vi "Transmitter_Monokrom_Mei - Copy.vi"() -> ()   [LabVIEW 2018]
uses:
  <vilib>/picture/picture.llb/imagedata.ctl
  <instrlib>/niUSRP/niUSRP Write Tx Data (CDB Cluster).vi
panel:
  out "size(s) 6":i32[](array[numeric])
  out "size(s) 5":i32
  out "IQ":i32
  out "R":i32
  out "output diterima":bool[][](array[boolean])
  out "Gambar Terima":picture
  in  "Width":i32=256
  in  "Height":i32=256
  out "unsigned 8bit integer":u8
  out "Array 2":i32[](array[numeric])
  out "size(s) 4":i32[](array[numeric])
  out "Array":i32[](array[numeric])
  out "output array 2":i16[][](array[numeric])
  out "output frame awal":i32[](array[numeric])
  out "subarray":i16[](array[numeric])
  in  "array":i32[](array[numeric])
  out "iterasi":i32
  out "hasil bagi":i32
  out "sisa bagi":i32
  out "size(s) 3":i32[](array[numeric])
  out "size(s) 2":i32
  out "size(s)":i32[](array[numeric])
  out "output array":i16[](array[numeric])
  in  "bit length":i32=3600
  out "x-y*floor(x/y)":i32
  out "output cluster 2":cluster{"t0":dbl, "dt":dbl, "Y":cdb[]}
  out "error out 2":errorcluster
  out "Frame Duration 2":dbl format="%#_6p"
  out "Waveform Graph 2":cluster{"t0":dbl, "dt":dbl, "Y":dbl[]}(graph)
  out "output":i16[](array[numeric])
  out "0, 1":i16[][](array[numeric])
  out "1-bit pixmap":bool[][](array[boolean])
  out "new picture":picture
  out "image data":T1
  in  "path to BMP file":path=path "D:/Thesis Pak Pri/pict.bmp"
  out "bits":i32[](array[numeric])
  in  "Modulation parameter":T2
  out "Bits length":i32
  out "USRP CoercedParamters":T3={"coerced IQ rate"=100000.0, "coerced carrier frequency"=100000.0, "coerced gain"=0.0} {"coerced gain" format="%#_6f"; "coerced carrier frequency" format="%#_6p"; "coerced IQ rate" format="%#_6p"}
  in  "error in (no error)":errorcluster
  in  "USRP ControledParameters":T4={"active antenna"="TX1", "gain"=0.0, "carrier frequency"=915000000.0, "IQ rate"=1000000.0} {"IQ rate" format="%#_6p"; "carrier frequency" format="%#_6p"; "gain" format="%#_6f"}
  in  "device names":refnum<k15>="192.168.10.1"
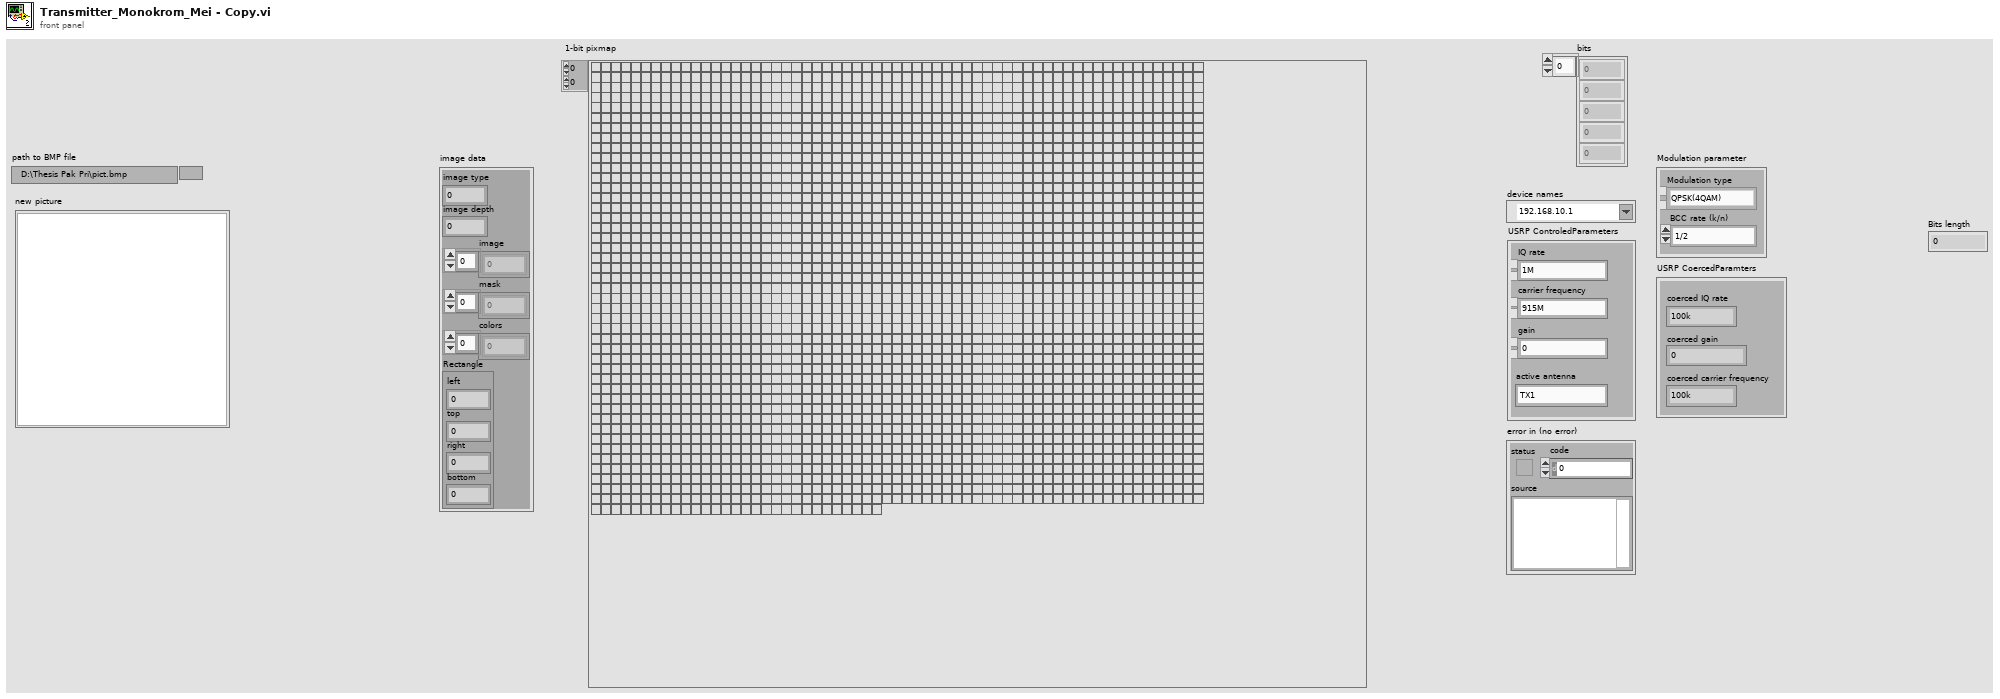
[diagram p1: front panel]
types:
  T1 = typedef "imagedata.ctl" = cluster{"image type":i32, "image depth":i32, "image":u8[], "mask":u8[], "colors":u32[], "Rectangle":cluster{"left":i16, "top":i16, "right":i16, "bottom":i16}}
  T2 = cluster{"Modulation type":enum16{"QPSK(4QAM)", "64QAM", "16QAM", "BPSK"}, "BCC rate (k/n)":enum16{"1/2", "2/3", "3/4"}}
  T3 = cluster{"coerced IQ rate":dbl, "coerced carrier frequency":dbl, "coerced gain":dbl}
  T4 = cluster{"active antenna":string, "gain":dbl, "carrier frequency":dbl, "IQ rate":dbl}
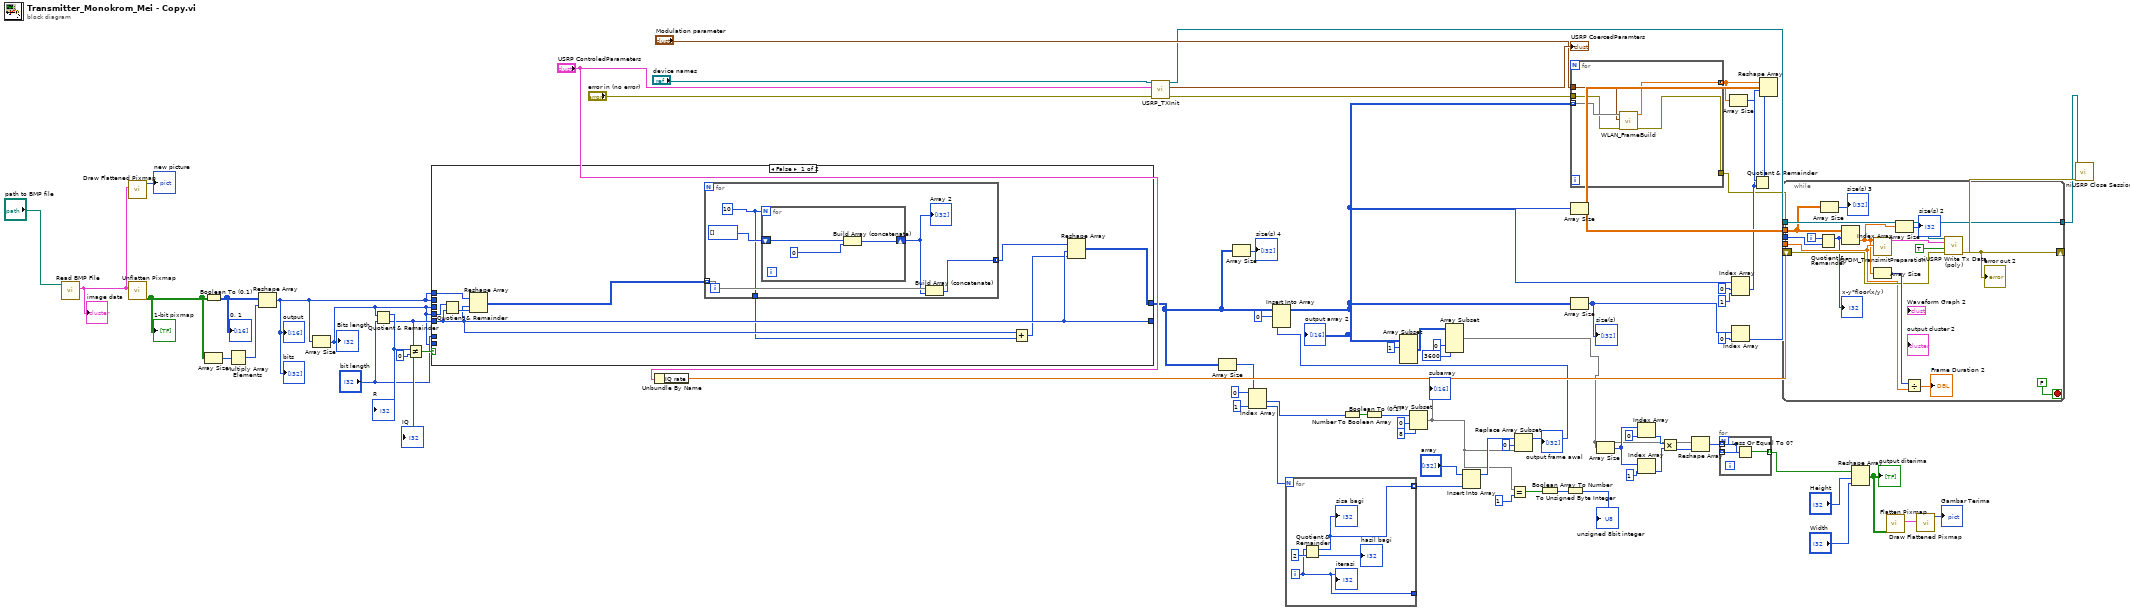
[diagram p0: block diagram]
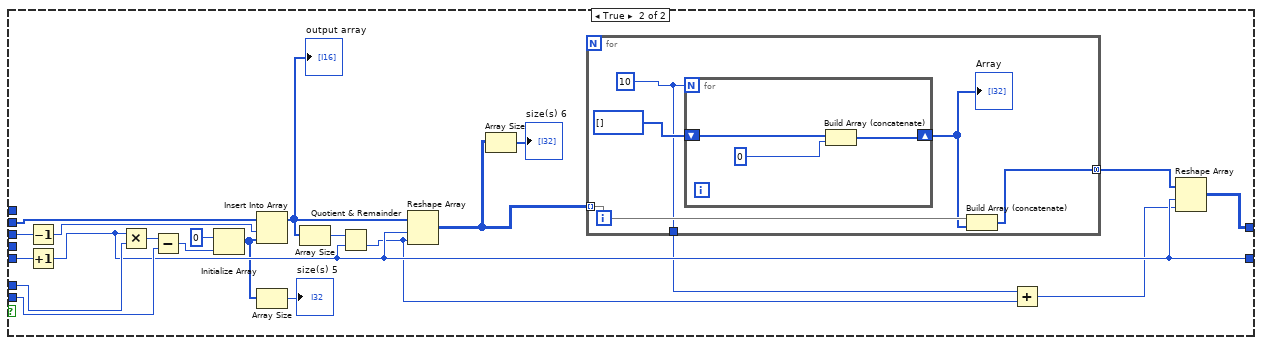
[diagram p2: hidden frame]
diagram:
  n1 = call <vilib>:"Read BMP File.vi"("path to BMP file"="path to BMP file") -> ("image data"=w71:T1)  [unwired: 8 in, 2 out]
  "image data" <- w71
  n2 = call <vilib>:"Draw Flattened Pixmap.vi"("image data"=w71) -> ("new picture"=→"new picture":picture)  [unwired: 8 in]
  n3 = call <vilib>:"Unflatten Pixmap.vi"("image data"=w71) -> ("1-bit pixmap"=w69:bool[][])  [unwired: 4 in, 6 out]
  "1-bit pixmap" <- w69
  n4 = Boolean To (0,1)(Boolean=w69) -> (0, 1=w2:i16[][])
  "0, 1" <- w2
  n5 = Array Size(array=w69) -> (size(s)=w70:i32[])
  n6 = Multiply Array Elements(1:w70) -> (0:w68:i32)
  n7 = Reshape Array(w2, w68) -> (w61:i16[])
  "bits" <- w61
  "output" <- w61
  n8 = Array Size(array=w61) -> (size(s)=w62:i32)
  "Bits length" <- w62
  n9 = Quotient & Remainder(x=w62, y="bit length") -> (x-y*floor(x/y)=w67:i32, floor(x/y)=w64:i32)
  "R" <- w67
  "IQ" <- w64
  n10 = Not Equal?(x=w67, y=0) -> (x != y?=w65:bool)
  n11 = case shown="False" w65 {
    tunnel: w64 -> [w81 w115]
    tunnel: "bit length" -> [_ w114]
    tunnel: w62 -> [_ w105]
    tunnel: w61 -> [_ w111]
    tunnel: w62 -> [_ w110]
    tunnel: [w81 w103] -> _
    tunnel: [w78 w99] -> w27
    tunnel: w62 -> [w85 _]
    tunnel: w61 -> [w86 _]
    frame False {
      n12 = Quotient & Remainder(x=w85, y=w81) -> (floor(x/y)=w84:i32)  [unwired: 1 out]
      n13 = Reshape Array(w86, w81, w84) -> (w83:i16[][])
      n14 = for {
        tunnel: w83 -> [w90] mode=indexing
        tunnel: [w88] -> w82 mode=concatenating
        tunnel: [w87] -> w80
        w87 = 10
        n15 = for {
          N: w87 -> [_]
          shift-right: [w92] -> w89
          shift-left: i32[] [] -> [w94]
          n16 = Build Array (concatenate)(w94, 0) -> (w92:i32[])
        }
        "Array 2" <- w89
        n17 = Build Array (concatenate)(w90, w89) -> (w88:i32[])
      }
      n18 = Add(x=w81, y=w80) -> (x+y=w79:i32)
      n19 = Reshape Array(w82, w81, w79) -> (w78:i32[][])
    }
    frame True {
      n20 = Decrement(x=w110) -> (x-1=w109:i32)
      n21 = Increment(x=w115) -> (x+1=w103:i32)
      n22 = Multiply(x=w103, y=w114) -> (x*y=w106:i32)
      n23 = Subtract(x=w106, y=w105) -> (x-y=w112:i32)
      n24 = Initialize Array(0 ("element"), w112) -> (w98:i32[])
      n25 = Insert Into Array(array=w111, index=w109, new element=w98) -> (w108:i16[])
      "output array" <- w108
      n26 = Array Size(array=w98) -> (size(s)=→"size(s) 5":i32)
      n27 = Array Size(array=w108) -> (size(s)=w107:i32)
      n28 = Quotient & Remainder(x=w107, y=w103) -> (floor(x/y)=w101:i32)  [unwired: 1 out]
      n29 = Reshape Array(w108, w103, w101) -> (w95:i16[][])
      n30 = Array Size(array=w95) -> (size(s)=→"size(s) 6":i32[])
      n31 = for {
        tunnel: w95 -> [w119] mode=indexing
        tunnel: [w116] -> w104 mode=concatenating
        tunnel: [w118] -> w102
        w118 = 10
        n32 = for {
          N: w118 -> [_]
          shift-right: [w121] -> w117
          shift-left: i32[] [] -> [w123]
          n33 = Build Array (concatenate)(w123, 0) -> (w121:i32[])
        }
        "Array" <- w117
        n34 = Build Array (concatenate)(w119, w117) -> (w116:i32[])
      }
      n35 = Add(x=w102, y=w101) -> (x+y=w100:i32)
      n36 = Reshape Array(w104, w103, w100) -> (w99:i32[][])
    }
  }
  n37 = Unbundle By Name("USRP ControledParameters") -> ("IQ rate"=w50:dbl)
  n38 = call "USRP_TXInit.vi"("device names"="device names", "USRP ControledParameters"="USRP ControledParameters", "error in (no error)"="error in (no error)") -> ("session handle out"=w49:refnum<k15>, "USRP CoercedParamters"=→"USRP CoercedParamters":T3, "error out"=w59:errorcluster)  [unwired: 5 in]
  n39 = Array Size(array=w27) -> (size(s)=w39:i32[])
  n40 = Array Size(array=w27) -> (size(s)=→"size(s) 4":i32[])
  n41 = Index Array(array=w39, index #1=0 ("index"), index #2=1 ("index")) -> (element #1=w35:i32, element #2=w36:i32)
  n42 = for {
    N: w36 -> [_]
    tunnel: [w125] -> _
    tunnel: [w124] -> w40 mode=indexing
    i -> [w125]
    n43 = Quotient & Remainder(x=w125, y=2) -> (x-y*floor(x/y)=w124:i32, floor(x/y)=→"hasil bagi":i32)
    "sisa bagi" <- w124
    "iterasi" <- w125
  }
  n44 = Number To Boolean Array(number=w35) -> (Boolean array=w42:bool[])
  n45 = Boolean To (0,1)(Boolean=w42) -> (0, 1=w33:i16[])
  n46 = Array Subset(array=w33, index=0, length=8) -> (w21:i16[])
  "subarray" <- w21
  n47 = Insert Into Array(array="array", new element=w40) -> (w30:i32[])  [unwired: 1 in]
  n48 = Equal?(x=w21, y=1) -> (x = y?=w24:bool[])
  n49 = Replace Array Subset(array=w30, new element=w21, index=0) -> (w28:i32[])
  "output frame awal" <- w28
  n50 = Insert Into Array(array=w27, index (row)=0, new element=w28) -> (w7:i32[][])  [unwired: 1 in]
  "output array 2" <- w7
  n51 = Array Subset(array=w7, index (row)=1 ("index")) -> (w5:i32[][])  [unwired: 3 in]
  n52 = Array Subset(array=w5, index (col)=0 ("index"), length (col)=3600 ("length")) -> (w1:i32[][])  [unwired: 2 in]
  n53 = Boolean Array To Number(Boolean array=w24) -> (number=w23:u32)
  n54 = To Unsigned Byte Integer(number=w23) -> (unsigned 8bit integer=→"unsigned 8bit integer":u8)
  n55 = for {
    tunnel: w7 -> [w132] mode=indexing
    tunnel: "Modulation parameter" -> [w129]
    tunnel: w59 -> [w128]
    tunnel: [w131] -> w47 mode=concatenating
    tunnel: [w130] -> w43
    n56 = call "WLAN_FrameBuild.vi"("error in (no error)"=w128, "Modulation parameter"=w129, "data in"=w132) -> ("error out"=w130:errorcluster, "output array"=w131:cdb[])  [unwired: 7 in]
  }
  n57 = Array Size(array=w7) -> (size(s)=w58:i32[])
  n58 = Array Size(array=w7) -> (size(s)=w53:i32[])
  "size(s)" <- w53
  n59 = Array Size(array=w1) -> (size(s)=w10:i32[])
  n60 = Index Array(array=w10, index=1) -> (element=w11:i32)
  n61 = Index Array(array=w10, index=0) -> (element=w12:i32)
  n62 = Multiply(x=w12, y=w11) -> (x*y=w9:i32)
  n63 = Reshape Array(w1, w9) -> (w8:i32[])
  n64 = for {
    tunnel: [w133] -> _ mode=indexing
    tunnel: [w134] -> w16 mode=indexing
    tunnel: [w133] -> _ mode=indexing
    tunnel: w8 -> [w133] mode=indexing
    n65 = Less Or Equal To 0?(x=w133) -> (x <= 0?=w134:bool)
  }
  n66 = Array Size(array=w47) -> (size(s)=w46:i32)
  n67 = Index Array(array=w58, index #1=0 ("index"), index #2=1 ("index")) -> (element #1=w45:i32)  [unwired: 1 out]
  n68 = Index Array(array=w53, index=0) -> (element=w51:i32)
  n69 = Quotient & Remainder(x=w46, y=w45) -> (floor(x/y)=w44:i32)  [unwired: 1 out]
  n70 = Reshape Array(w47, w45, w44) -> (w54:cdb[][])
  n71 = while {
    tunnel: w54 -> [w136]
    tunnel: w50 -> [w144]
    shift-right: [w145] -> w55
    shift-left: w43 -> [w146]
    tunnel: w49 -> [w139]
    tunnel: w51 -> [w140]
    tunnel: [w139] -> w48
    i -> [w143]
    stop <- FALSE stop-if-true
    n72 = Quotient & Remainder(x=w143, y=w140) -> (x-y*floor(x/y)=w142:i32)  [unwired: 1 out]
    "x-y*floor(x/y)" <- w142
    n73 = Array Size(array=w136) -> (size(s)=→"size(s) 3":i32[])
    n74 = Index Array(array=w136, index (row)=w142) -> (element=w138:cdb[])  [unwired: 1 in]
    n75 = call "OFDM_TransimitPreparation.vi"("IQ rate"=w144, "array"=w138) -> ("output cluster"=w149:cluster{"t0":dbl, "dt":dbl, "Y":cdb[]})  [unwired: 9 in]
    n76 = Array Size(array=w138) -> (size(s)=w150:i32)
    n77 = Array Size(array=w138) -> (size(s)=→"size(s) 2":i32)
    n78 = Divide(x=w150, y=w144) -> (x/y=→"Frame Duration 2":dbl)
    n79 = call-poly <instrlib>:"niUSRP Write Tx Data (poly).vi"("session handle"=w139, "data"=w149, "end of data?"=TRUE, "error in (no error)"=w146) -> ("error out"=w145:errorcluster)  [unwired: 10 in, 1 out]
    "error out 2" <- w145
  }
  n80 = Reshape Array(w16, "Height", "Width") -> (w15:bool[][])
  "output diterima" <- w15
  n81 = call <vilib>:"Flatten Pixmap.vi"("1-bit pixmap"=w15) -> ("image data"=w18:T1)  [unwired: 10 in]
  n82 = call <vilib>:"Draw Flattened Pixmap.vi"("image data"=w18) -> ("new picture"=→"Gambar Terima":picture)  [unwired: 8 in]
  n83 = call <instrlib>:"niUSRP Close Session.vi"("session handle"=w48, "error in (no error)"=w55) -> ()  [unwired: 13 in, 1 out]
